vi "Get Images.vi"(8 "error in":errorcluster, 11 "Stop (F)":bool) -> (0 "error out":errorcluster, 1 "Left Image out":T1, 2 "Right Image out":T1, 3 "Gauge":cluster{dbl, dbl}(knob) scale=0.0..50.0)   [LabVIEW 2012]
uses:
  <vilib>/vision/Image Controls.llb/IMAQ Image.ctl
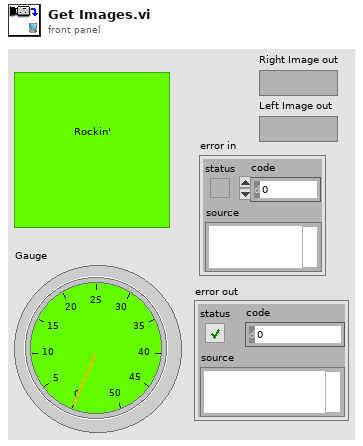
[diagram p1: front panel]
types:
  T1 = typedef "IMAQ Image.ctl" = refnum<image>
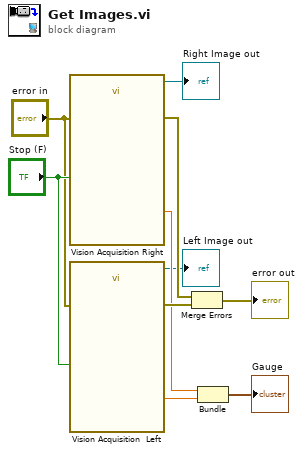
[diagram p0: block diagram]
diagram:
  n1 = call "Vision Acquisition Right"("Stop (F)"="Stop (F)", "error in"="error in") -> ("Image Out"=→"Right Image out":T1, "Frame Rate"=w7:dbl, "error out"=w10:errorcluster)  [unwired: 21 in, 2 out]
  n2 = call "Vision Acquisition  Left"("Stop (F)"="Stop (F)", "error in"="error in") -> ("Image Out"=→"Left Image out":T1, "Frame Rate"=w6:dbl, "error out"=w9:errorcluster)  [unwired: 21 in, 2 out]
  n3 = Merge Errors(w10, w9) -> (→"error out":errorcluster)
  n4 = Bundle("Frame Rate"=w7, "Frame Rate"=w6) -> (→"Gauge":cluster{"Frame Rate":dbl, "Frame Rate":dbl})  [unwired: 1 in]
